vi "Update Status Channels.vi"(8 "error in (no error)":errorcluster, 10 "DMA Input Settings":T1[](array[typedef]) {"DMA Settings"."dt" format="%#_p"; "DMA Settings"."Update Rate" items=["1 Hz"=1, "2 Hz"=2, "5 Hz"=5, "10 Hz"=10]; "Write to VS Engine.Refs"."Refs" format="%.0x"}, 11 "DMA Output Settings":T6[](array[typedef]) {"Write to VS Engine.Refs"."Refs" format="%.0x"}) -> (0 "error out":errorcluster, 2 "DMA Input Settings":T1[](array[typedef]) {"DMA Settings"."dt" format="%#_p"; "DMA Settings"."Update Rate" items=["1 Hz"=1, "2 Hz"=2, "5 Hz"=5, "10 Hz"=10]; "Write to VS Engine.Refs"."Refs" format="%.0x"}, 3 "DMA Output Settings":T6[](array[typedef]) {"Write to VS Engine.Refs"."Refs" format="%.0x"})   [LabVIEW 2013, in "FPGA Addon Engine.lvlib"]
uses:
  FPGA Addon Engine.lvlib
  Types/DMA Output References.ctl
  <vilib>/NI Veristand/Custom Device API/Data Reference.ctl
  <vilib>/NI Veristand/Custom Device Waveform API/Single Waveform Read (DBL)/Single Waveform Read (DBL).lvclass
  Types/DMA Output Ref.ctl
  Types/DMA Input References.ctl
  <vilib>/NI Veristand/Custom Device Waveform API/Multiple Waveforms Write (DBL)/Multiple Waveforms Write (DBL).lvclass
  Types/DMA Input Ref.ctl
  Shared/DMA Settings.ctl
  Shared/Delacing Scheme.ctl
  <vilib>/NI Veristand/Custom Device API/NI VeriStand - Set Channel Value by Data Reference.vi
  <vilib>/NI Veristand/Custom Device API/Global Data Refs.vi
  Inline Async API/Inline Async API.lvlib
  <vilib>/NI VeriStand/Custom Device API/Custom Device API.lvlib
  Shared/FPGA Addon Shared.lvlib
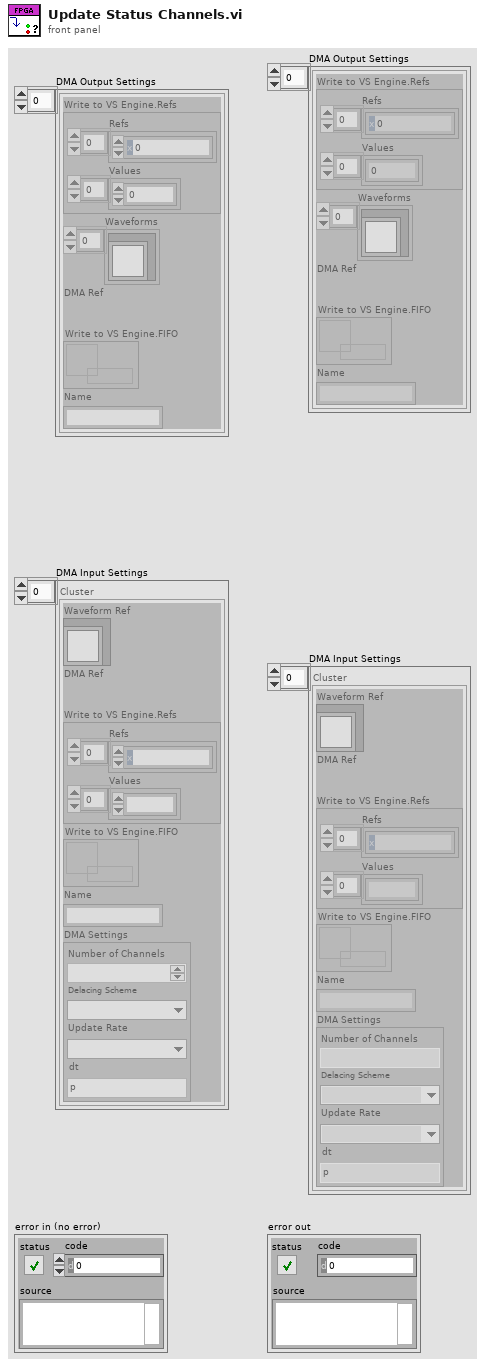
[diagram p1: front panel]
types:
  T1 = typedef "FPGA Addon Engine.lvlib/DMA Input References.ctl" = cluster{"Waveform Ref":refnum<class "Multiple Waveforms Write (DBL).lvclass">, "DMA Ref":T2, "Write to VS Engine.Refs":cluster{"Refs":T3[], "Values":dbl[]}, "Write to VS Engine.FIFO":refnum<k33>, "Name":string, "DMA Settings":T4}
  T2 = typedef "FPGA Addon Engine.lvlib/DMA Input Ref.ctl" = refnum<k20>
  T3 = typedef "Custom Device API.lvlib/Data Reference.ctl" = i32
  T4 = typedef "FPGA Addon Shared.lvlib/DMA Settings.ctl" = cluster{"Number of Channels":u8, "Delacing Scheme":T5, "Update Rate":u32, "dt":dbl}
  T5 = typedef "FPGA Addon Shared.lvlib/Delacing Scheme.ctl" = enum8{"Interlaced"}
  T6 = typedef "FPGA Addon Engine.lvlib/DMA Output References.ctl" = cluster{"Write to VS Engine.Refs":cluster{"Refs":T3[], "Values":dbl[]}, "Waveforms":refnum<class "Single Waveform Read (DBL).lvclass">[], "DMA Ref":T7, "Write to VS Engine.FIFO":refnum<k33>, "Name":string}
  T7 = typedef "FPGA Addon Engine.lvlib/DMA Output Ref.ctl" = refnum<k20>
  T8 = cluster{"Chan Refs":T3[], "Previous Chan Values":dbl[]}
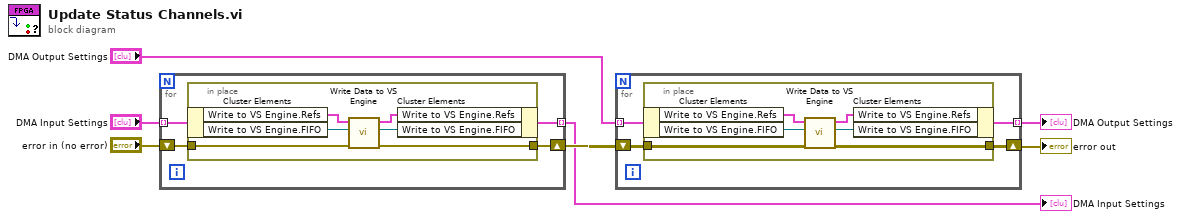
[diagram p0: block diagram]
diagram:
  n1 = for {
    shift-right: [w10] -> w6
    shift-left: "error in (no error)" -> [w11]
    tunnel: "DMA Input Settings" -> [w9] mode=indexing
    tunnel: [w8] -> w3 mode=indexing
    n2 = in-place {
      in-place-border: w11 -> [w16]
      in-place-border: [w15] -> w10
      n3 = in-place-cluster #1(w9) -> ("Write to VS Engine.Refs"=w14:cluster{"Refs":T3[], "Values":dbl[]}, "Write to VS Engine.FIFO"=w13:refnum<k33>)
      n4 = call "Write Data to VS Engine.vi"("error in"=w16, "Write to VS Engine FIFO"=w13, "Channel Pairs"=w14) -> ("error out"=w15:errorcluster, "Channel Pairs Out"=w12:T8)  [unwired: 6 in, 1 out]
      n5 = in-place-cluster #1("Write to VS Engine.Refs"=w12, "Write to VS Engine.FIFO"=w13) -> (w8:T1)
    }
  }
  "DMA Input Settings" <- w3
  n6 = for {
    shift-right: [w19] -> w7
    shift-left: w6 -> [w20]
    tunnel: "DMA Output Settings" -> [w18] mode=indexing
    tunnel: [w17] -> w5 mode=indexing
    n7 = in-place {
      in-place-border: w20 -> [w25]
      in-place-border: [w24] -> w19
      n8 = in-place-cluster #2(w18) -> ("Write to VS Engine.Refs"=w23:cluster{"Refs":T3[], "Values":dbl[]}, "Write to VS Engine.FIFO"=w22:refnum<k33>)
      n9 = call "Write Data to VS Engine.vi"("error in"=w25, "Write to VS Engine FIFO"=w22, "Channel Pairs"=w23) -> ("error out"=w24:errorcluster, "Channel Pairs Out"=w21:T8)  [unwired: 6 in, 1 out]
      n10 = in-place-cluster #2("Write to VS Engine.Refs"=w21, "Write to VS Engine.FIFO"=w22) -> (w17:T6)
    }
  }
  "error out" <- w7
  "DMA Output Settings" <- w5
